vi "EventStructure.vi"() -> ()   [LabVIEW 2019]
panel:
  in  "stop 2":bool
  out "Count":u32
  in  "Increment":bool
  in  "stop":bool
  out "Count":u32
  in  "Increment Number":bool
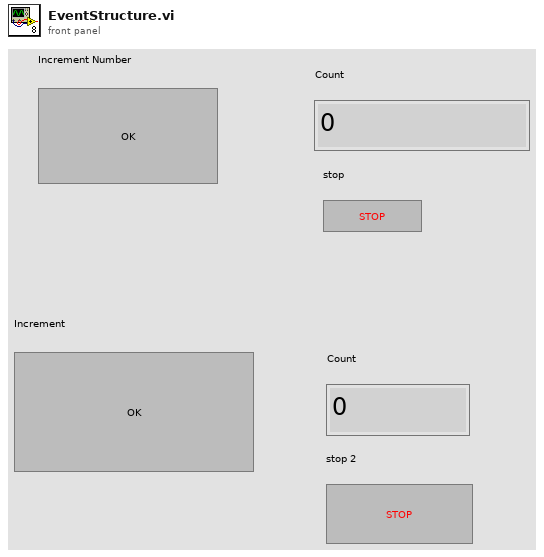
[diagram p1: front panel]
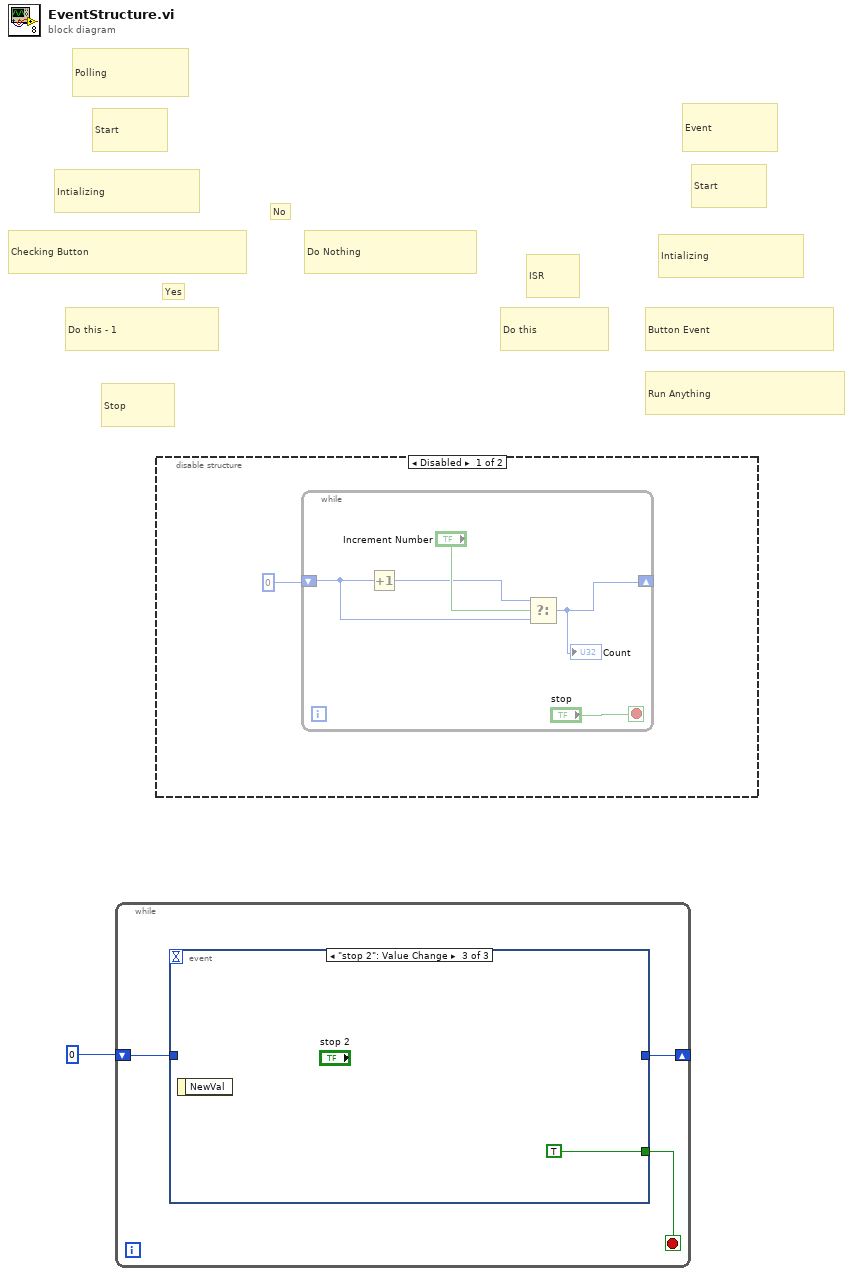
[diagram p0: block diagram]
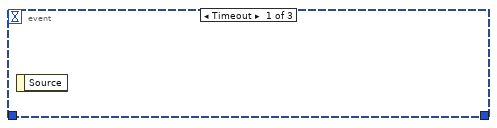
[diagram p2: hidden frame]
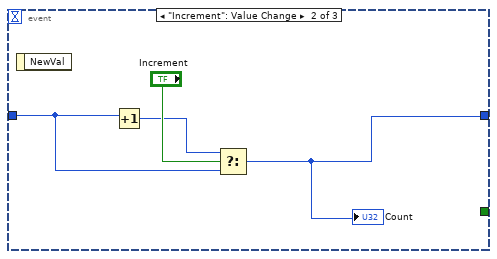
[diagram p3: hidden frame]
diagram:
  # "Run Anything"
  # "ISR"
  # "Do this"
  # "Button Event"
  # "Event"
  # "Intializing"
  # "Start"
  # "Polling"
  # "Yes"
  # "No"
  # "Stop"
  # "Do Nothing"
  # "Do this - 1"
  # "Checking Button"
  # "Intializing"
  # "Start"
  n1 = while {
    shift-right: [w3] -> _
    shift-left: u32 0 ("Count") -> [w4]
    stop <- w2 stop-if-true
    n2 = event shown="[2] \"stop 2\": Value Change" {
      selector: _ -> [_ _ _]
      dyn-events: _ -> [_ _ _]
      timeout: _ -> [_ _ _]
      tunnel: w4 -> [_ w6 _]
      tunnel: [_ w5 _] -> w3
      tunnel: [_ _ TRUE] -> w2
      event Timeout {
        n3 = event-data() -> ()  [unwired: 1 in, 1 out]
      }
      event "Increment": Value Change {
        n4 = event-data() -> ()  [unwired: 1 in, 1 out]
        n5 = Increment(x=w6) -> (x+1=w7:u32)
        n6 = Select(t=w7, s="Increment", f=w6) -> (s? t:f=w5:u32)
        "Count" <- w5
      }
      event "stop 2": Value Change {
        n7 = event-data() -> ()  [unwired: 1 in, 1 out]
      }
    }
  }
  n8 = disable-structure shown="Disabled" {
    frame Disabled {
      n9 = while {
        shift-right: [w12] -> _
        shift-left: u32 0 ("Count") -> [w13]
        stop <- "stop" stop-if-true
        n10 = Increment(x=w13) -> (x+1=w14:u32)
        n11 = Select(t=w14, s="Increment Number", f=w13) -> (s? t:f=w12:u32)
        "Count" <- w12
      }
    }
    frame Enabled {
    }
  }
